vi "Display Item in Tree.vi"(4 "Condensed?":bool=TRUE, 5 "Item Name":string, 7 "Parent Tag":string, 8 "error in (no error)":errorcluster, 10 "Data":variant, 11 "Tree Refnum":refnum<vi>) -> (0 "error out":errorcluster, 3 "Tree Refnum out":refnum<vi>)   [LabVIEW 2015, in "YAML Parser.lvclass"]
uses:
  YAML Parser.lvclass
  <vilib>/ErrorRing/Error Ring.xnode
  <vilib>/Utility/Data Type/NI_Data Type.lvlib
  <vilib>/Utility/error.llb/whitespace.ctl
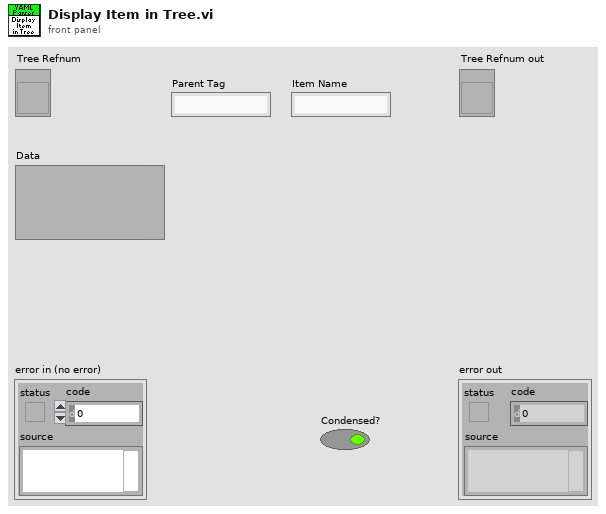
[diagram p1: front panel]
types:
  T1 = typedef "NI_Data Type.lvlib/Data Type.ctl" = enum8{"Invalid Type", "Void", "I8", "I16", "I32", "I64", "U8", "U16", "U32", "U64", "Single Float", "Double Float", "Extended Float", "Single Complex", "Double Complex", "Extended Complex", "Enum U8", "Enum U16", "Enum U32", "Enum U64", "Single Float With Unit", "Double Float With Unit", "Extended Float With Unit", "Single Complex with Unit", "Double Complex with Unit", "Extended Complex with Unit", "Boolean", "String", "Path", "Picture", "Tag", "Array", "Cluster", "Variant", "LV Variant", "Waveform", "Timestamp", "Digital Waveform", "Digital Data", "ExpressData", "Refnum", "External Data", "VI", "Poly VI", "LabVIEW Class Instance", "Fixed Point"}
  T2 = typedef "whitespace.ctl" = u16
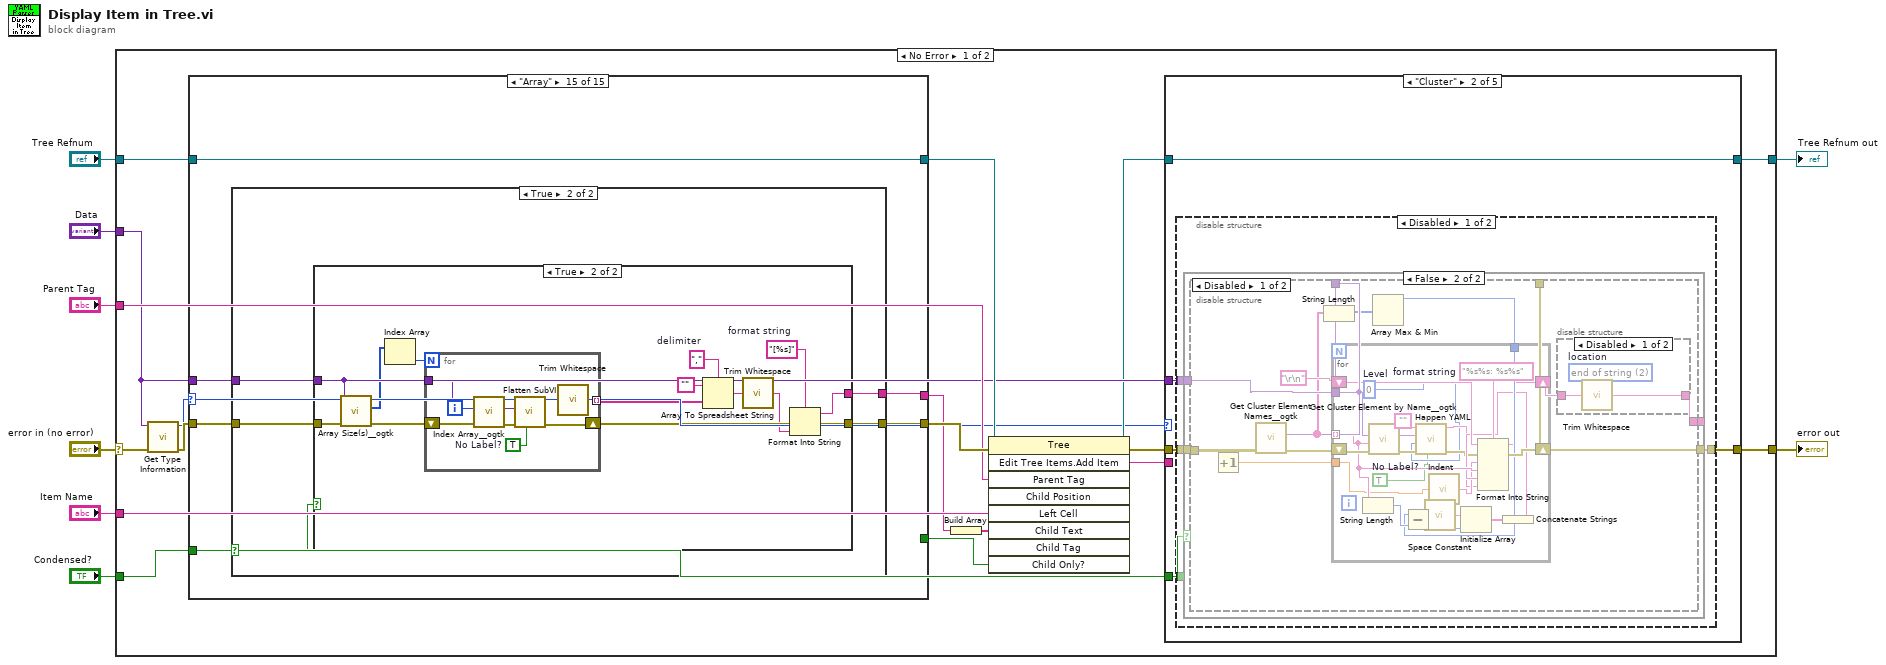
[diagram p0: block diagram]
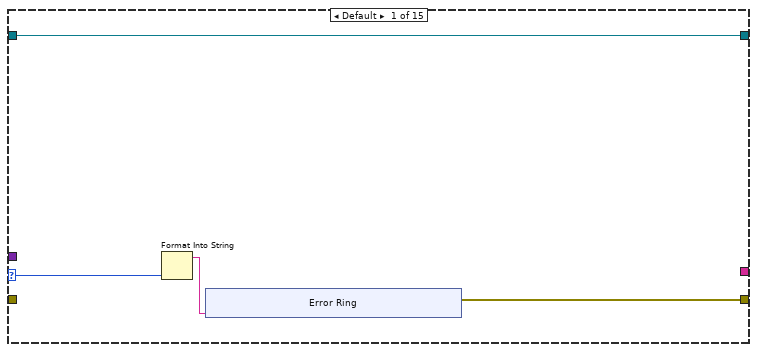
[diagram p2: hidden frame]
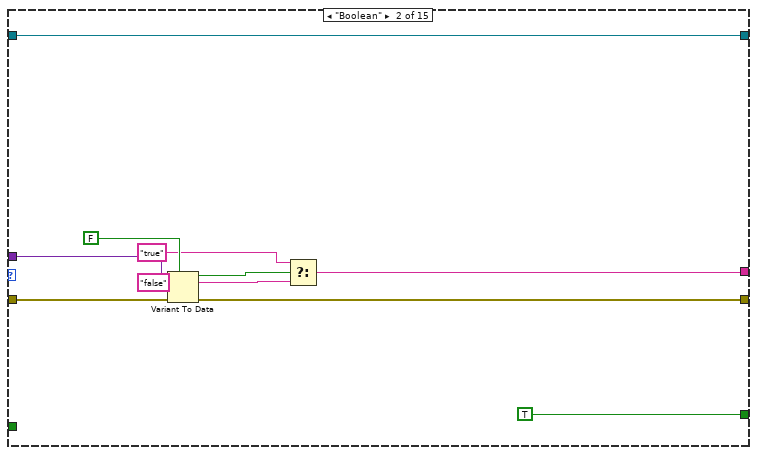
[diagram p3: hidden frame]
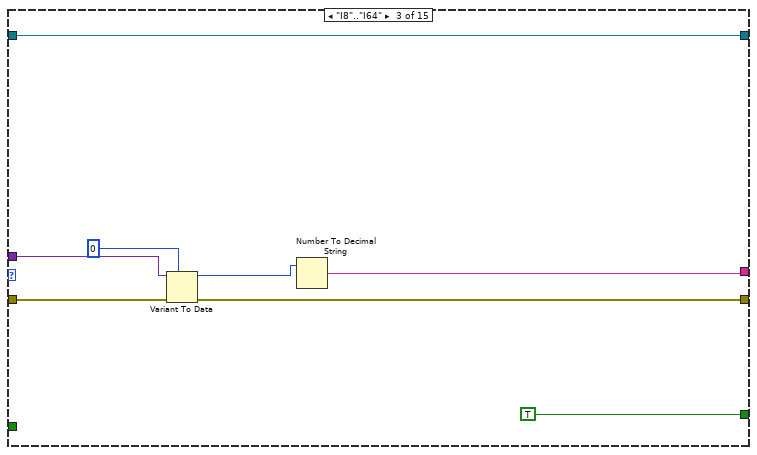
[diagram p4: hidden frame]
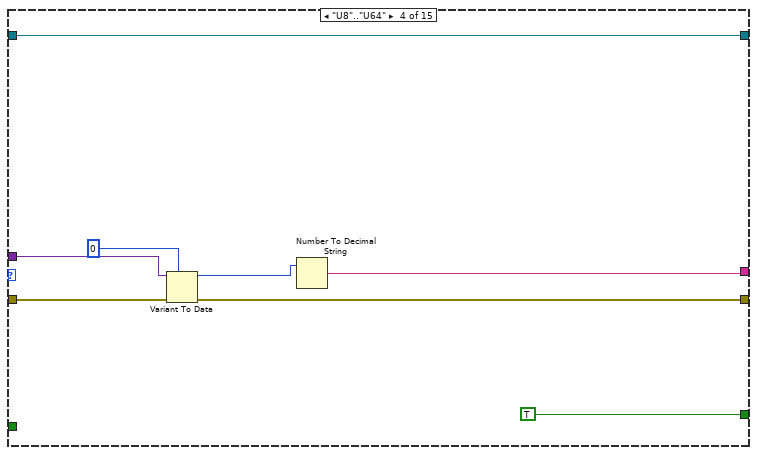
[diagram p5: hidden frame]
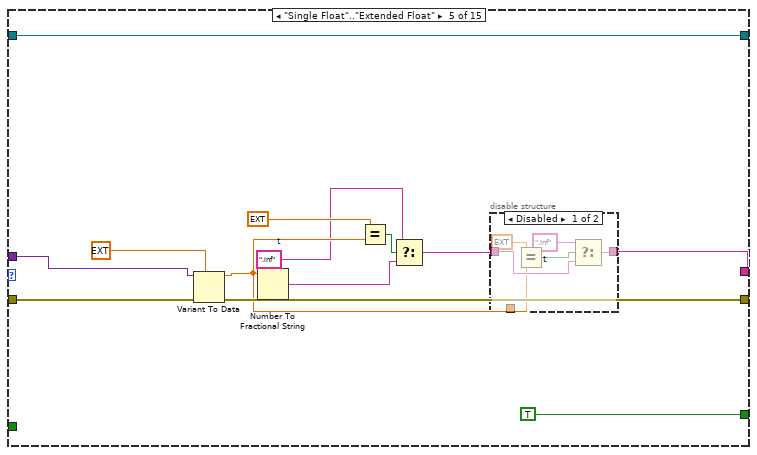
[diagram p6: hidden frame]
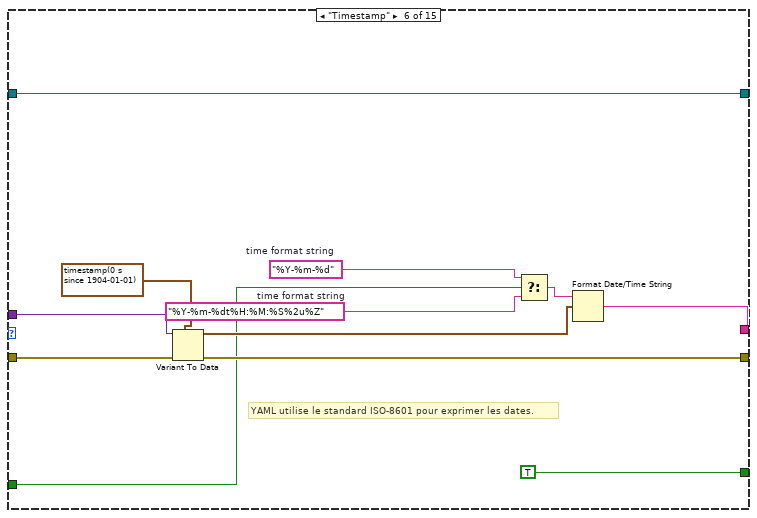
[diagram p8: hidden frame]
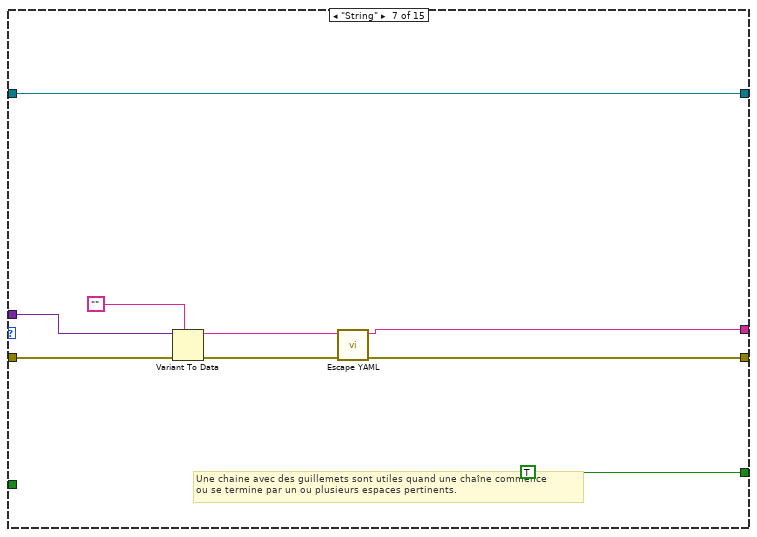
[diagram p9: hidden frame]
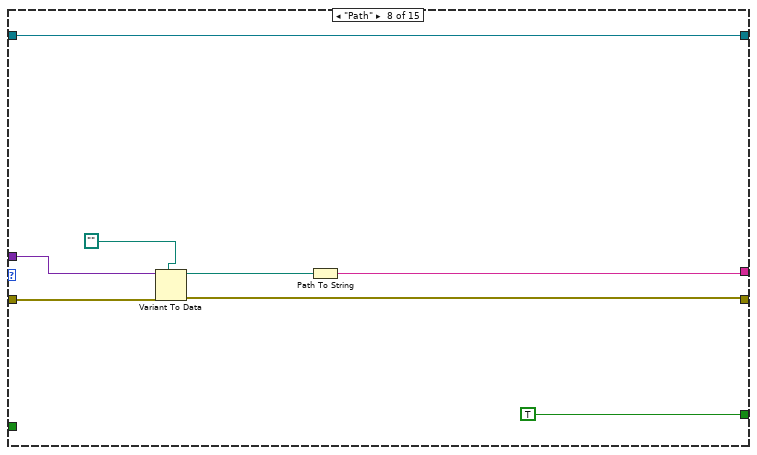
[diagram p10: hidden frame]
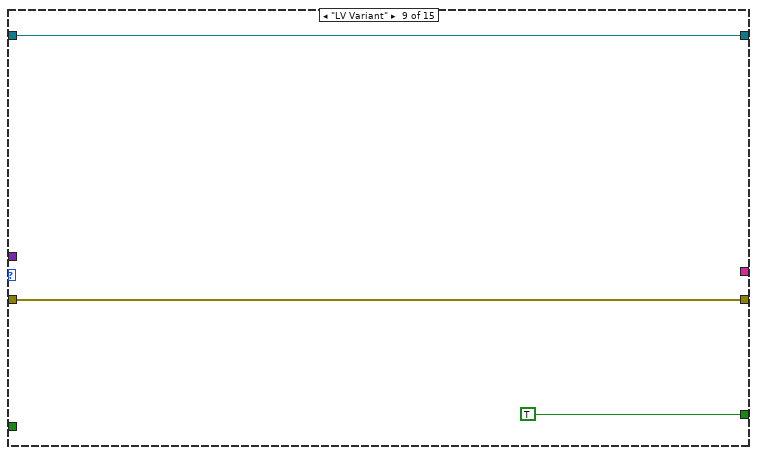
[diagram p11: hidden frame]
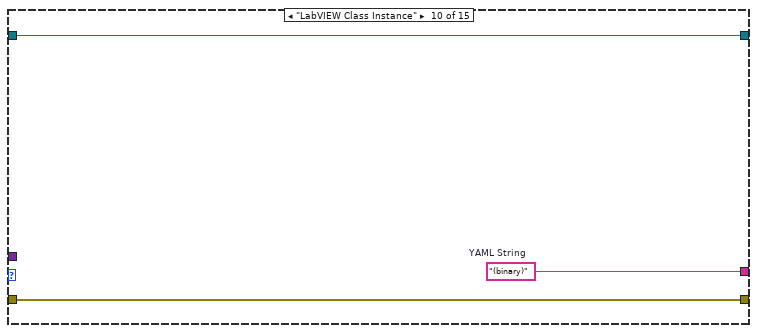
[diagram p12: hidden frame]
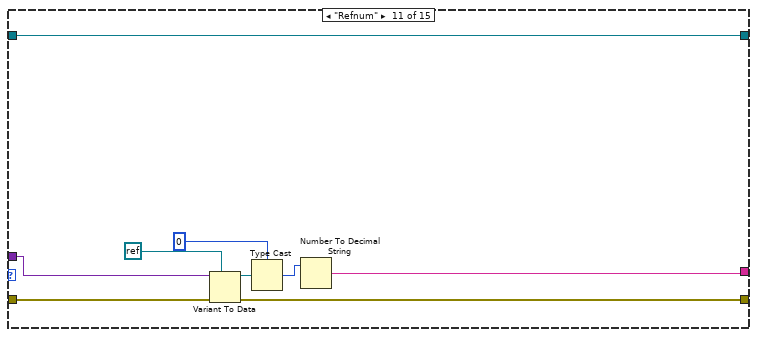
[diagram p13: hidden frame]
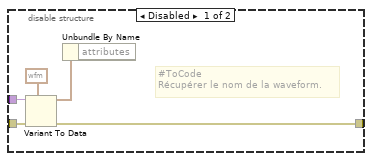
[diagram p15: hidden frame]
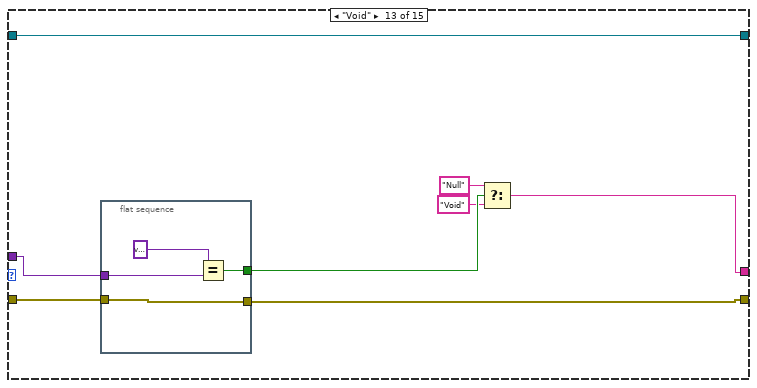
[diagram p16: hidden frame]
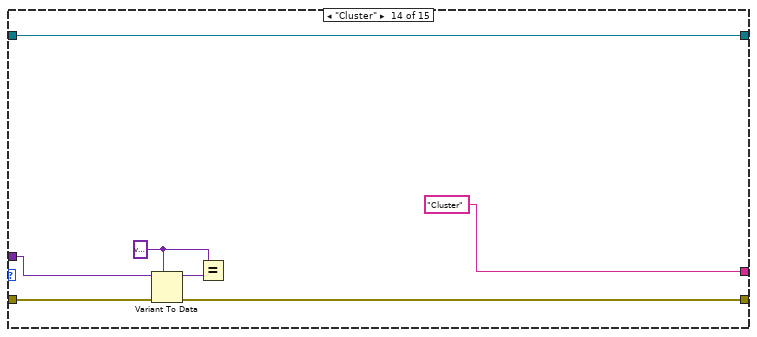
[diagram p17: hidden frame]
diagram:
  n1 = case shown="No Error" "error in (no error)" {
    selector: "error in (no error)" -> [w26 w354]
    tunnel: [w15 w354] -> w7
    tunnel: [w11 w353] -> w4
    tunnel: "Tree Refnum" -> [w20 w353]
    tunnel: "Condensed?" -> [w9 _]
    tunnel: "Data" -> [w13 _]
    tunnel: "Parent Tag" -> [w23 _]
    tunnel: "Item Name" -> [w19 _]
    frame No Error {
      n2 = call <vilib>:"Get Type Information.vi"("error in (no error)"=w26, "Variant"=w13) -> ("error out"=w25:errorcluster, "Type"=w10:T1)  [unwired: 5 in, 3 out]
      n3 = case shown="\"Array\"" w10 {
        selector: w10 -> [w27 _ _ _ _ _ _ _ _ _ _ _ _ _ _]
        tunnel: w25 -> [_ w45 w53 w61 w74 w93 w101 w110 w113 w115 w120 w128 w136 w153 w158]
        tunnel: w13 -> [_ w44 w52 w60 w73 w92 w100 w109 _ _ w119 w127 w138 w148 w156]
        tunnel: [w28 w42 w50 w58 w71 w89 w96 w105 w113 w115 w117 w126 w137 w152 w157] -> w24
        tunnel: [_ w38 w48 w56 w64 w88 w95 w106 _ w114 w118 _ w139 "Cluster" ("YAML String") w155] -> w18
        tunnel: w9 -> [_ _ _ _ _ w87 _ _ _ _ _ _ _ _ w159]
        tunnel: [_ TRUE TRUE TRUE TRUE TRUE TRUE TRUE TRUE _ _ _ _ _ _] -> w22
        tunnel: [w30 w36 w46 w54 w62 w82 w98 w103 w111 w116 w125 w129 w143 w154 w160] -> w21
        tunnel: w20 -> [w30 w36 w46 w54 w62 w82 w98 w103 w111 w116 w125 w129 w143 w154 w160]
        frame Default {
          n4 = Format Into String(w27) -> (resulting string=w29:string)  [unwired: 3 in, 1 out]
          n5 = xnode "Error Ring"("parameter 0"=w29) -> ("error out"=w28:errorcluster)
        }
        frame "Boolean" {
          n6 = Variant To Data(error in=w45, type=FALSE, Variant=w44) -> (data=w41:bool, error out=w42:errorcluster)
          n7 = Select(t="true", s=w41, f="false") -> (s? t:f=w38:string)
        }
        frame "I8".."I64" {
          n8 = Variant To Data(error in=w53, type=i64 0, Variant=w52) -> (data=w49:i64, error out=w50:errorcluster)
          n9 = Number To Decimal String(number=w49) -> (decimal integer string=w48:string)  [unwired: 1 in]
        }
        frame "U8".."U64" {
          n10 = Variant To Data(error in=w61, type=u64 0, Variant=w60) -> (data=w57:u64, error out=w58:errorcluster)
          n11 = Number To Decimal String(number=w57) -> (decimal integer string=w56:string)  [unwired: 1 in]
        }
        frame "Single Float".."Extended Float" {
          w65 = ".inf"  # t
          n12 = Variant To Data(error in=w74, type=ext 0.0, Variant=w73) -> (data=w66:ext, error out=w71:errorcluster)
          n13 = Number To Fractional String(number=w66) -> (F-format string=w68:string)  [unwired: 3 in]
          n14 = Equal?(x=ext inf, y=w66) -> (x = y?=w69:bool)
          n15 = Select(t=w65, s=w69, f=w68) -> (s? t:f=w67:string)
          n16 = disable-structure shown="Disabled" {
            disable-tunnel: w67 -> [w78 w81]
            disable-tunnel: w66 -> [w77 _]
            disable-tunnel: [w75 w81] -> w64
            frame Disabled {
              w76 = ".inf"  # t
              n17 = Equal?(x=ext -inf, y=w77) -> (x = y?=w79:bool)
              n18 = Select(t=w76, s=w79, f=w78) -> (s? t:f=w75:string)
            }
            frame Enabled {
            }
          }
        }
        frame "Timestamp" {
          w85 = "%Y-%m-%d"  # time format string
          w86 = "%Y-%m-%dt%H:%M:%S%2u%Z"  # time format string
          # "YAML utilise le standard ISO-8601 pour exprimer les dates."
          n19 = Variant To Data(error in=w93, type=timestamp(0 s since 1904-01-01), Variant=w92) -> (data=w90:timestamp, error out=w89:errorcluster)
          n20 = Select(t=w85, s=w87, f=w86) -> (s? t:f=w84:string)
          n21 = Format Date/Time String(time format string (%c)=w84, seconds (now)=w90) -> (date/time string=w88:string)  [unwired: 1 in]
        }
        frame "String" {
          # "Une chaine avec des guillemets sont utiles quand une chaîne commence \nou se termine par un ou plusieurs espaces pertinents."
          n22 = Variant To Data(error in=w101, type="", Variant=w100) -> (data=w94:string, error out=w97:errorcluster)
          n23 = call "Escape YAML.vi"("error in (no error)"=w97, "String"=w94) -> ("error out"=w96:errorcluster, "YAML String"=w95:string)  [unwired: 8 in]
        }
        frame "Path" {
          n24 = Variant To Data(error in=w110, type=path "", Variant=w109) -> (data=w107:path, error out=w105:errorcluster)
          n25 = Path To String(path=w107) -> (string=w106:string)
        }
        frame "LV Variant" {
        }
        frame "LabVIEW Class Instance" {
          w114 = "(binary)"  # YAML String
        }
        frame "Refnum" {
          n26 = Variant To Data(error in=w120, type=refnum<k0> refnum, Variant=w119) -> (data=w122:refnum<k0>, error out=w117:errorcluster)
          n27 = Type Cast(type=u32 0, x=w122) -> (*(type *) &x=w121:u32)
          n28 = Number To Decimal String(number=w121) -> (decimal integer string=w118:string)  [unwired: 1 in]
        }
        frame "Waveform" {
          n29 = disable-structure shown="Enabled" {
            disable-tunnel: w128 -> [w134 w135]
            disable-tunnel: w127 -> [w133 _]
            disable-tunnel: [w130 w135] -> w126
            frame Disabled {
              # "#ToCode\nRécupérer le nom de la waveform."
              n30 = Variant To Data(error in=w134, type=waveform(dbl) {"t0"=timestamp(0 s since 1904-01-01), "dt"=1.0, "Y"=[]} ("Waveform"), Variant=w133) -> (data=w131:waveform(dbl), error out=w130:errorcluster)
              n31 = Unbundle By Name(w131) -> ()  [unwired: 1 out]
            }
            frame Enabled {
            }
          }
        }
        frame "Void" {
          n32 = flat-sequence {
            tunnel: [w146] -> w142
            tunnel: w138 -> [w145]
            tunnel: [w144] -> w137
            tunnel: w136 -> [w144]
            frame #0 {
              n33 = Equal?(x=variant, y=w145) -> (x = y?=w146:bool)
            }
          }
          n34 = Select(t="Null" ("YAML String"), s=w142, f="Void" ("YAML String")) -> (s? t:f=w139:string)
        }
        frame "Cluster" {
          w150 = variant
          n35 = Variant To Data(error in=w153, type=w150, Variant=w148) -> (data=w151:variant, error out=w152:errorcluster)
          n36 = Equal?(x=w150, y=w151) -> ()  [unwired: 1 out]
        }
        frame "Array" {
          n37 = case shown="True" w159 {
            selector: w159 -> [_ w162]
            tunnel: w158 -> [w161 w166]
            tunnel: [w161 w164] -> w157
            tunnel: w156 -> [_ w165]
            tunnel: [_ w163] -> w155
            frame False {
            }
            frame True {
              n38 = case shown="True" w162 {
                tunnel: w166 -> [w167 w177]
                tunnel: w165 -> [_ w176]
                tunnel: [w167 w174] -> w164
                tunnel: [_ w173] -> w163
                frame False {
                }
                frame True {
                  w169 = "[%s]"  # format string
                  w172 = ","  # delimiter
                  n39 = call <userlib>:"Array Size(s)__ogtk.vi"("error in (no error)"=w177, "Array"=w176) -> ("error out"=w179:errorcluster, "Size(s)"=w181:u32[])  [unwired: 7 in, 1 out]
                  n40 = Index Array(array=w181) -> (element=w180:u32)  [unwired: 1 in]
                  n41 = for {
                    N: w180 -> [_]
                    shift-right: [w185] -> w175
                    shift-left: w179 -> [w190]
                    tunnel: w176 -> [w189]
                    tunnel: [w187] -> w178 mode=indexing
                    i -> [w188]
                    w184 = TRUE  # No Label?
                    n42 = call <userlib>:"Index Array__ogtk.vi"("error in (no error)"=w190, "Index (1D)"=w188, "MultiD Array"=w189) -> ("error out"=w186:errorcluster, "Array Element"=w182:variant)  [unwired: 7 in]
                    n43 = call "Flatten SubVI.vi"("No Label?"=w184, "error in (no error)"=w186, "Data"=w182) -> ("error out"=w185:errorcluster, "YAML String out"=w183:string)  [unwired: 7 in]
                    n44 = call <vilib>:"Trim Whitespace.vi"("string"=w183) -> ("trimmed string"=w187:string)  [unwired: 1 in]
                  }
                  n45 = Array To Spreadsheet String(delimiter (Tab)=w172, array=w178, 3:"") -> (spreadsheet string=w171:string)
                  n46 = call <vilib>:"Trim Whitespace.vi"("string"=w171) -> ("trimmed string"=w168:string)  [unwired: 1 in]
                  n47 = Format Into String(format string=w169, error in=w175, w168) -> (resulting string=w173:string, error out=w174:errorcluster)  [unwired: 1 in]
                }
              }
            }
          }
        }
      }
      n48 = Build Array(w18) -> (w17:string[])
      n49 = invoke class="Tree" method="Edit Tree Items.Add Item"(reference=w21, error in=w24, "Parent Tag"=w23, "Left Cell"=w19, "Child Text"=w17, "Child Only?"=w22) -> (reference out=w12:refnum<vi>, error out=w16:errorcluster, "Edit Tree Items:Add Item"=w14:string)  [unwired: 3 in, 6 out]
      n50 = case shown="\"Cluster\"" w10 {
        tunnel: w16 -> [w191 w196 w277 w294 w335]
        tunnel: w13 -> [_ w195 w276 w293 w334]
        tunnel: [w191 w197 w278 w295 w330] -> w15
        tunnel: w9 -> [_ w194 w275 w292 _]
        tunnel: [w192 w193 w273 w291 w331] -> w11
        tunnel: w12 -> [w192 w193 w274 w290 w332]
        tunnel: w14 -> [_ _ w272 w289 w325]
        frame Default {
        }
        frame "Cluster" {
          n51 = disable-structure shown="Disabled" {
            disable-tunnel: [w201 w268] -> w197
            disable-tunnel: w196 -> [w200 w268]
            disable-tunnel: w195 -> [w199 _]
            disable-tunnel: w194 -> [w198 _]
            frame Disabled {
              n52 = case shown="False" w198 {
                tunnel: [w217 w230] -> w201
                tunnel: w200 -> [w215 w229]
                tunnel: w199 -> [w213 w228]
                tunnel: [w203 w227] -> _
                frame True {
                  w209 = ","  # delimiter
                  # "{ PHP: 5.2, MySQL: 5.1, Apache: 2.2.20 }"
                  n53 = Increment() -> (x+1=w216:dbl)  [unwired: 1 in]
                  n54 = call <userlib>:"Get Cluster Element Names__ogtk.vi"("error in (no error)"=w215, "Cluster"=w213) -> ("error out"=w214:errorcluster, "Element Names"=w212:string[])  [unwired: 8 in]
                  n55 = String Length(string=w212) -> (length=w211:i32[])
                  n56 = Array Max & Min(array=w211) -> (max value=w210:i32)  [unwired: 3 out]
                  n57 = for {
                    shift-right: [w221] -> w217
                    shift-left: w214 -> [w226]
                    tunnel: w216 -> [_]
                    tunnel: w212 -> [w224] mode=indexing
                    tunnel: w213 -> [w225]
                    tunnel: w210 -> [_]
                    tunnel: [w223] -> w205 mode=indexing
                    w219 = u32 0  # Level
                    n58 = call <userlib>:"Get Cluster Element by Name__ogtk.vi"("error in (no error)"=w226, "Element Name"=w224, "Cluster"=w225) -> ("error out"=w222:errorcluster, "VElement"=w218:variant)  [unwired: 6 in, 1 out]
                    n59 = call "Happen YAML.vi"("error in (no error)"=w222, "Level"=w219, "Anything"=w218) -> ("error out"=w221:errorcluster, "YAML String out"=w220:string)  [unwired: 7 in]
                    n60 = call <vilib>:"Trim Whitespace.vi"("string"=w220) -> ("trimmed string"=w223:string)  [unwired: 1 in]
                  }
                  n61 = Array To Spreadsheet String(delimiter (Tab)=w209, array=w205, 3:"") -> (spreadsheet string=w208:string)
                  n62 = call <vilib>:"Trim Whitespace.vi"("string"=w208) -> ("trimmed string"=w202:string)  [unwired: 1 in]
                  n63 = Concatenate Strings("{", w202, "}") -> (w203:string)
                }
                frame False {
                  n64 = disable-structure shown="Disabled" {
                    disable-tunnel: [w241 _] -> w230
                    disable-tunnel: w229 -> [w237 _]
                    disable-tunnel: w228 -> [w235 _]
                    disable-tunnel: [w234 _] -> w227
                    frame Disabled {
                      n65 = Increment() -> (x+1=w238:dbl)  [unwired: 1 in]
                      n66 = call <userlib>:"Get Cluster Element Names__ogtk.vi"("error in (no error)"=w237, "Cluster"=w235) -> ("error out"=w236:errorcluster, "Element Names"=w233:string[])  [unwired: 8 in]
                      n67 = String Length(string=w233) -> (length=w232:i32[])
                      n68 = Array Max & Min(array=w232) -> (max value=w231:i32)  [unwired: 3 out]
                      n69 = for {
                        shift-right: [w265] -> w241
                        shift-left: w236 -> [w267]
                        shift-right: [w255] -> w239
                        shift-left: "\r\n" -> [w264]
                        tunnel: w238 -> [w254]
                        tunnel: w233 -> [w262] mode=indexing
                        tunnel: w235 -> [w266]
                        tunnel: w231 -> [w260]
                        w248 = u32 0  # Level
                        w263 = "%s%s: %s%s"  # format string
                        w246 = TRUE  # No Label?
                        n70 = String Length(string=w262) -> (length=w261:i32)
                        n71 = call <userlib>:"Get Cluster Element by Name__ogtk.vi"("error in (no error)"=w267, "Element Name"=w262, "Cluster"=w266) -> ("error out"=w252:errorcluster, "VElement"=w249:variant)  [unwired: 6 in, 1 out]
                        n72 = Subtract(x=w260, y=w261) -> (x-y=w257:i32)
                        n73 = call "Happen YAML.vi"("No Label?"=w246, "error in (no error)"=w252, "Level"=w248, "Anything"=w249, "YAML String in"="") -> ("error out"=w251:errorcluster, "YAML String out"=w250:string)  [unwired: 5 in]
                        n74 = call <vilib>:"Space Constant.vi"() -> ("String"=w259:string)
                        n75 = call "Indent.vi"("Index"=w254) -> ("Indentation"=w253:string)
                        n76 = Initialize Array(w259, w257) -> (w258:string[])
                        n77 = Concatenate Strings(w258) -> (w256:string)
                        n78 = Format Into String(format string=w263, initial string=w264, error in=w251, w253, w262, w256, w250) -> (resulting string=w255:string, error out=w265:errorcluster)
                      }
                      n79 = disable-structure shown="Disabled" {
                        disable-tunnel: w239 -> [w244 w245]
                        disable-tunnel: [w243 w245] -> w234
                        frame Disabled {
                          w242 = T2 2 items=["both", "start of string", "end of string"]  # location
                          n80 = call <vilib>:"Trim Whitespace.vi"("string"=w244, "location (both)"=w242) -> ("trimmed string"=w243:string)
                        }
                        frame Enabled {
                        }
                      }
                    }
                    frame Enabled {
                    }
                  }
                }
              }
            }
            frame Enabled {
            }
          }
        }
        frame "Void" {
          n81 = Get Variant Attribute(Variant=w276, error in=w277) -> (duplicate Variant=w269:variant, names=w270:string[], error out=w271:errorcluster)  [unwired: 2 in, 1 out]
          n82 = for {
            shift-right: [w285] -> w278
            shift-left: w271 -> [w287]
            tunnel: w270 -> [w279] mode=indexing
            tunnel: w269 -> [w288]
            tunnel: w275 -> [w284]
            shift-right: [w282] -> w273
            shift-left: w274 -> [w283]
            tunnel: w272 -> [w280]
            n83 = Get Variant Attribute(Variant=w288, name=w279, error in=w287) -> (value=w281:variant, error out=w286:errorcluster)  [unwired: 1 in, 2 out]
            n84 = call "Display Item in Tree.vi"("Condensed?"=w284, "Item Name"=w279, "Parent Tag"=w280, "error in (no error)"=w286, "Data"=w281, "Tree Refnum"=w283) -> ("error out"=w285:errorcluster, "Tree Refnum out"=w282:refnum<vi>)  [unwired: 4 in]
          }
        }
        frame "Array" {
          n85 = case shown="False" w292 {
            tunnel: [w296 w306] -> w295
            tunnel: w294 -> [w296 w305]
            tunnel: w293 -> [_ w304]
            tunnel: [w297 w299] -> w291
            tunnel: w290 -> [w297 w300]
            tunnel: w289 -> [_ w298]
            frame True {
            }
            frame False {
              n86 = call <userlib>:"Array Size(s)__ogtk.vi"("error in (no error)"=w305, "Array"=w304) -> ("error out"=w301:errorcluster, "Size(s)"=w303:u32[])  [unwired: 7 in, 1 out]
              n87 = Index Array(array=w303) -> (element=w302:u32)  [unwired: 1 in]
              n88 = for {
                N: w302 -> [_]
                shift-right: [w314] -> w306
                shift-left: w301 -> [w319]
                tunnel: w304 -> [w318]
                shift-right: [w315] -> w299
                shift-left: w300 -> [w317]
                tunnel: w298 -> [w312]
                i -> [w311]
                n89 = call <userlib>:"Index Array__ogtk.vi"("error in (no error)"=w319, "Index (1D)"=w311, "MultiD Array"=w318) -> ("error out"=w316:errorcluster, "Array Element"=w313:variant)  [unwired: 7 in]
                n90 = Number To Decimal String(number=w311) -> (decimal integer string=w310:string)  [unwired: 1 in]
                n91 = Concatenate Strings("[" ("string"), w310, "]" ("string")) -> (w309:string)
                n92 = call "Display Item in Tree.vi"("Item Name"=w309, "Parent Tag"=w312, "error in (no error)"=w316, "Data"=w313, "Tree Refnum"=w317) -> ("error out"=w314:errorcluster, "Tree Refnum out"=w315:refnum<vi>)  [unwired: 5 in]
              }
            }
          }
        }
        frame "Waveform" {
          w320 = TRUE  # Condensed?
          n93 = Variant To Data(error in=w335, type=waveform(dbl) {"t0"=timestamp(0 s since 1904-01-01), "dt"=1.0, "Y"=[]} ("Waveform"), Variant=w334) -> (data=w337:waveform(dbl), error out=w333:errorcluster)
          n94 = Unbundle By Name(w337) -> ("t0"=w329:timestamp, "dt"=w328:dbl, "Y"=w327:dbl[], "attributes"=w326:variant)
          n95 = call "Display Item in Tree.vi"("Item Name"="t0", "Parent Tag"=w325, "error in (no error)"=w333, "Data"=w329, "Tree Refnum"=w332) -> ("error out"=w342:errorcluster, "Tree Refnum out"=w343:refnum<vi>)  [unwired: 5 in]
          n96 = call "Display Item in Tree.vi"("Item Name"="dt", "Parent Tag"=w325, "error in (no error)"=w342, "Data"=w328, "Tree Refnum"=w343) -> ("error out"=w340:errorcluster, "Tree Refnum out"=w341:refnum<vi>)  [unwired: 5 in]
          n97 = call "Display Item in Tree.vi"("Condensed?"=w320, "Item Name"="Y", "Parent Tag"=w325, "error in (no error)"=w340, "Data"=w327, "Tree Refnum"=w341) -> ("error out"=w338:errorcluster, "Tree Refnum out"=w339:refnum<vi>)  [unwired: 4 in]
          n98 = disable-structure shown="Disabled" {
            disable-tunnel: w339 -> [w350 w352]
            disable-tunnel: w338 -> [w349 w351]
            disable-tunnel: [w348 w352] -> w331
            disable-tunnel: [w347 w351] -> w330
            disable-tunnel: w326 -> [w346 _]
            disable-tunnel: w325 -> [w345 _]
            disable-tunnel: "attributes" ("Item Name") -> [w344 _]
            frame Disabled {
              n99 = call "Display Item in Tree.vi"("Item Name"=w344, "Parent Tag"=w345, "error in (no error)"=w349, "Data"=w346, "Tree Refnum"=w350) -> ("error out"=w347:errorcluster, "Tree Refnum out"=w348:refnum<vi>)  [unwired: 5 in]
            }
            frame Enabled {
            }
          }
        }
      }
    }
    frame Error {
    }
  }
  "error out" <- w7
  "Tree Refnum out" <- w4
